vi "Autonics_Hall_GMR_Vector_report2014.vi"() -> ()   [LabVIEW 2018]
uses:
  <vilib>/Platform/NI_3dgraph.lvlib
  <vilib>/Utility/file.llb/Write To Spreadsheet File (DBL).vi
  <vilib>/DAQmx/create/channels.llb/DAQmx Create Channel (DO-Digital Output).vi
  <vilib>/DAQmx/write.llb/DAQmx Write (Digital 1D Bool 1Chan 1Samp).vi
  <vilib>/DAQmx/read.llb/DAQmx Read (Analog 2D DBL NChan NSamp).vi
  <vilib>/DAQmx/configure/timing.llb/DAQmx Timing (Sample Clock).vi
  <vilib>/DAQmx/create/channels.llb/DAQmx Create Channel (AI-Voltage-Basic).vi
  <resource>/objmgr/daqmx.rc
  <vilib>/Math Plots/3D Math Plots/3D Quiver/3D Quiver Datatype/3D Quiver Datatype.lvclass
  <vilib>/Math Plots/3D Math Plots/3D Quiver/3D Quiver Datatype/Public/Plot Helper (Vector).vi
  <vilib>/Analysis/Matrix/NI_Matrix.lvlib
  <vilib>/Utility/file.llb/Read From Spreadsheet File (DBL).vi
  <vilib>/Analysis/Matrix/Numeric/Multiply/Multiply - R,RM.vi
  <vilib>/Analysis/Matrix/Numeric/Multiply/Multiply - RM,R.vi
  <vilib>/Math Plots/2D Math Plots/2D Feather/2D Feather Datatype/2D Feather Datatype.lvclass
  <vilib>/Math Plots/2D Math Plots/2D Feather/2D Feather Datatype/Public/Plot Helper (Vector).vi
  <vilib>/Instr/_visa.llb/VISA Configure Serial Port (Instr).vi
  <vilib>/Math Plots/3D Math Plots/3D Quiver/3D Quiver XCtrl/3D Quiver.xctl
  <vilib>/Math Plots/2D Math Plots/2D Feather/2D Feather XCtrl/2D Feather.xctl
panel:
  out "2D Feather":refnum<class "2D Plot Datatype.lvclass">[](xcontrol)
  in  "GMR":refnum<k7>(container)
  in  "Z Length":dbl=2.0
  in  "X Length":dbl=50.0
  out "X_Z_Scale":sgl=111.11112
  in  "Invert ?":bool
  out "Time Step":u32
  in  "Open":bool
  out "3D Vector":refnum<class "3D Plot Datatype.lvclass">[](xcontrol)
  in  "Scan Distance":dbl=50.0
  in  "Multiplier":dbl=10.0
  in  "Save Button":bool
  in  "No Save":bool
  in  "Save/Open Link":path
  in  "ViewMode":i32(ring) items=["cwViewXYPlane", "cwViewXZPlane", "cwViewYZPlane", "cwViewUserDefined"]
  in  "Back data":bool
  in  "Data Type":u16(ring) items=["Normal", "dX", "dY"]
  in  "Scan Channel":fxp<+,8,8>
  in  "Scan Channel Control":tag="Dev3/port0/line0:7"
  in  "Sampling Rate(Hz)":dbl=15000.0
  in  "Samples per Channels":i32=1000
  in  "Min Volts":dbl=-10.0 format="%0.2f"
  in  "Max Volts":dbl=10.0 format="%0.2f"
  in  "Channels":tag="Dev3/ai0:63"
  in  "Scan Step (mm)":dbl=1.0
  in  "Scan":bool
  in  "Plot style":i32(ring)=5 items=["cwLine"=1, "cwPoint"=2, "cwLinePoint"=3, "cwHiddenLine"=4, "cwSurface"=5, "cwSurfaceLine"=6, "cwSurfaceNormal"=7, "cwContourLine"=8, "cwSurfaceContour"=9]
  in  "Hall":refnum<k7>(container)
  in  "Flow control":u16(ring) items=["None", "XON/XOFF", "RTS/CTS", "XON/XOFF & RTS/CTS", "DTR/DSR", "XON/XOFF & DTR/DSR"]
  in  "Stop bits":u16(ring)=10 items=["1.0"=10, "1.5"=15, "2.0"=20]
  in  "Parity":dbl
  in  "Data bits":u16=8 min=5 max=8 step=1
  in  "Baud Rate":u32=57600
  in  "COM Port":refnum<visa-resource-name>="COM3"
  in  "Travel per Pulse (mm)":dbl=0.002
  in  "Speed (mm/s)":dbl=5.0
  out "Current  Position (mm)":dbl format="%#_4g"
  in  "Move Distance (mm)":dbl=1.0
  in  "Stop Scan":bool
  in  "Stop":bool
  in  "Home":bool
  in  "Right":bool
  in  "Left":bool
  # "SCANER CONTROL"
  # "CRACKS INSPECTION"
  # "COM Setting"
  # "CHANNELS"
  # "TIMING"
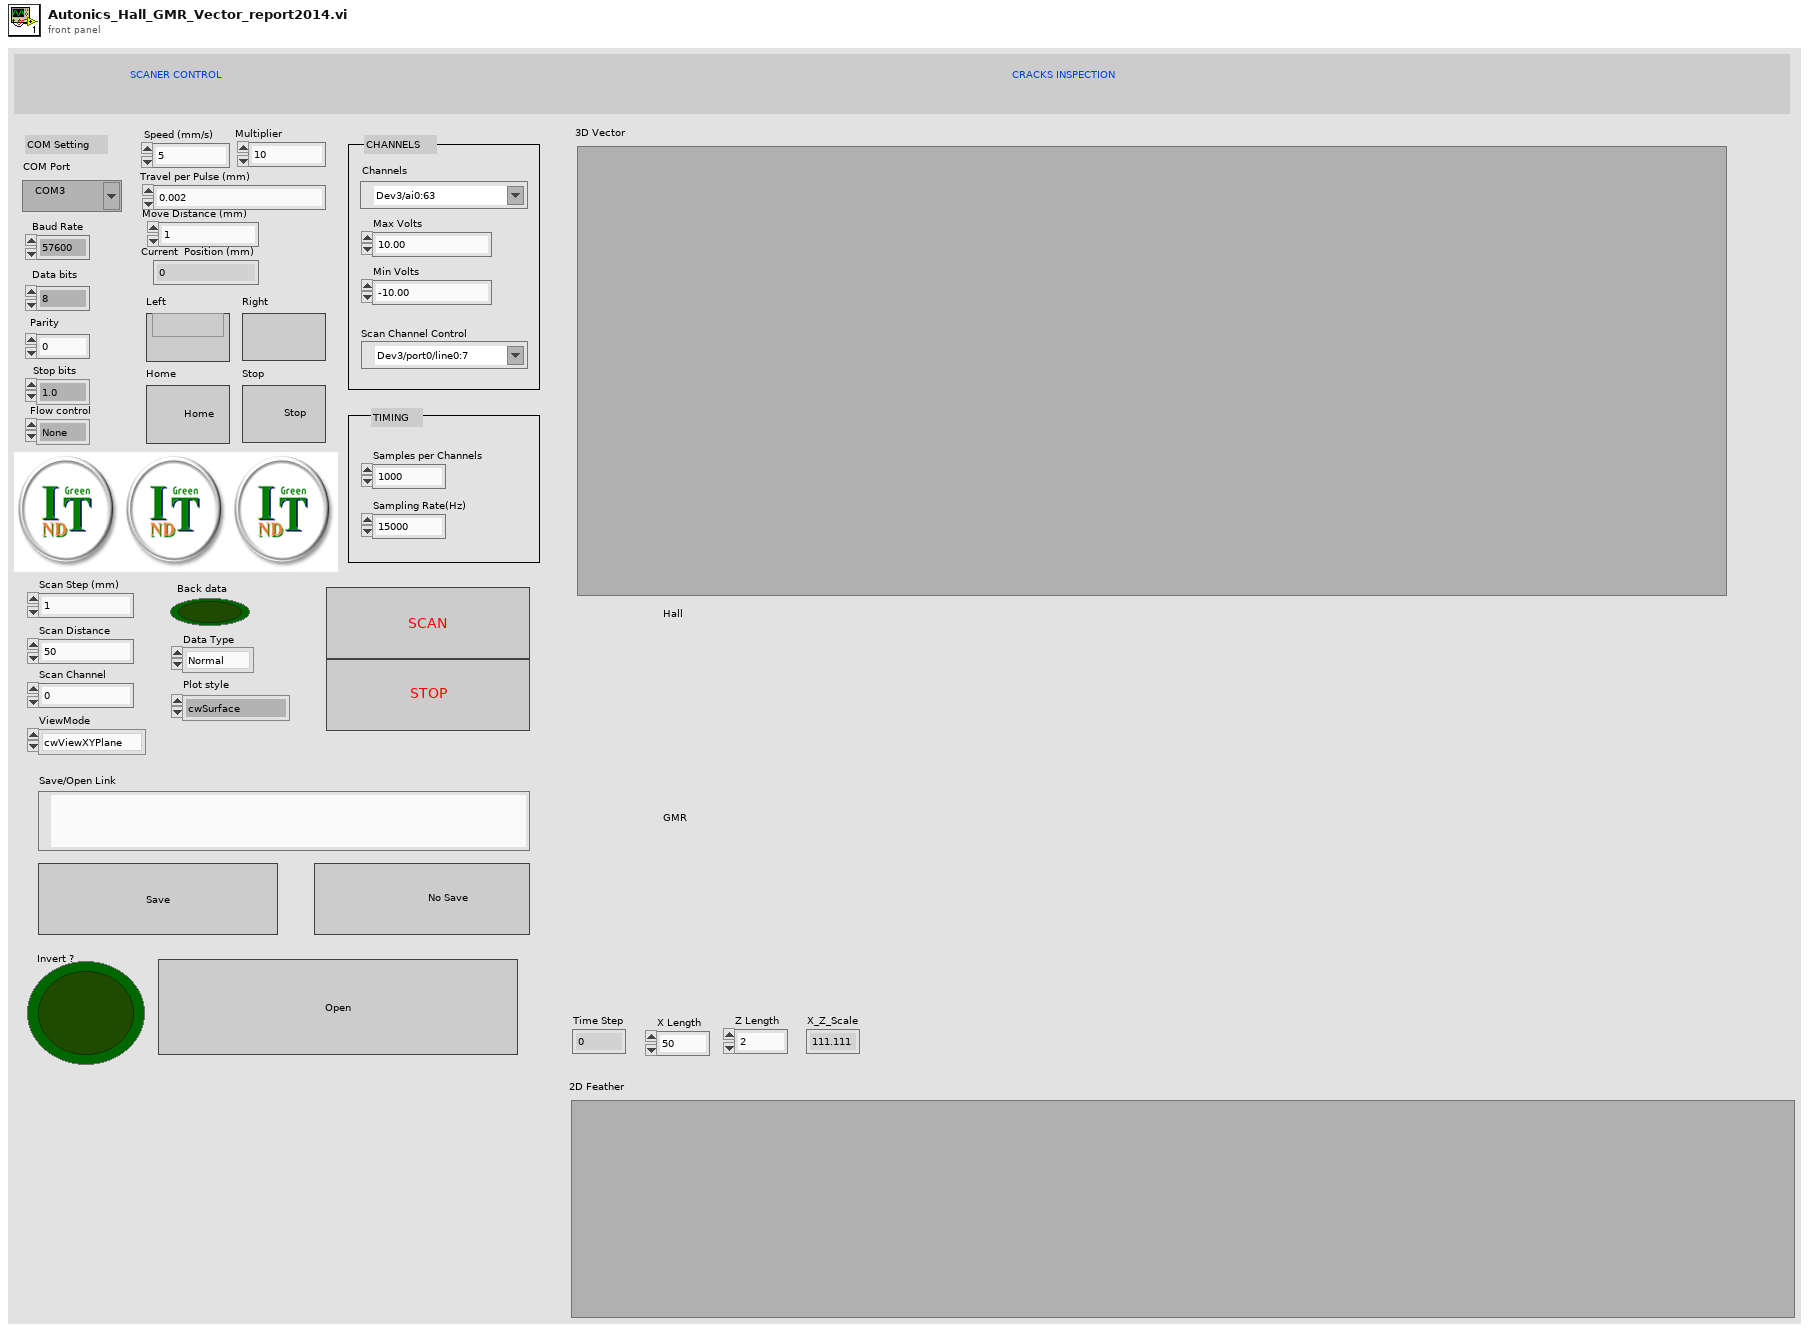
[diagram p1: front panel]
types:
  T1 = typedef "NI_Matrix.lvlib/RealMatrix.ctl" = dbl[][]
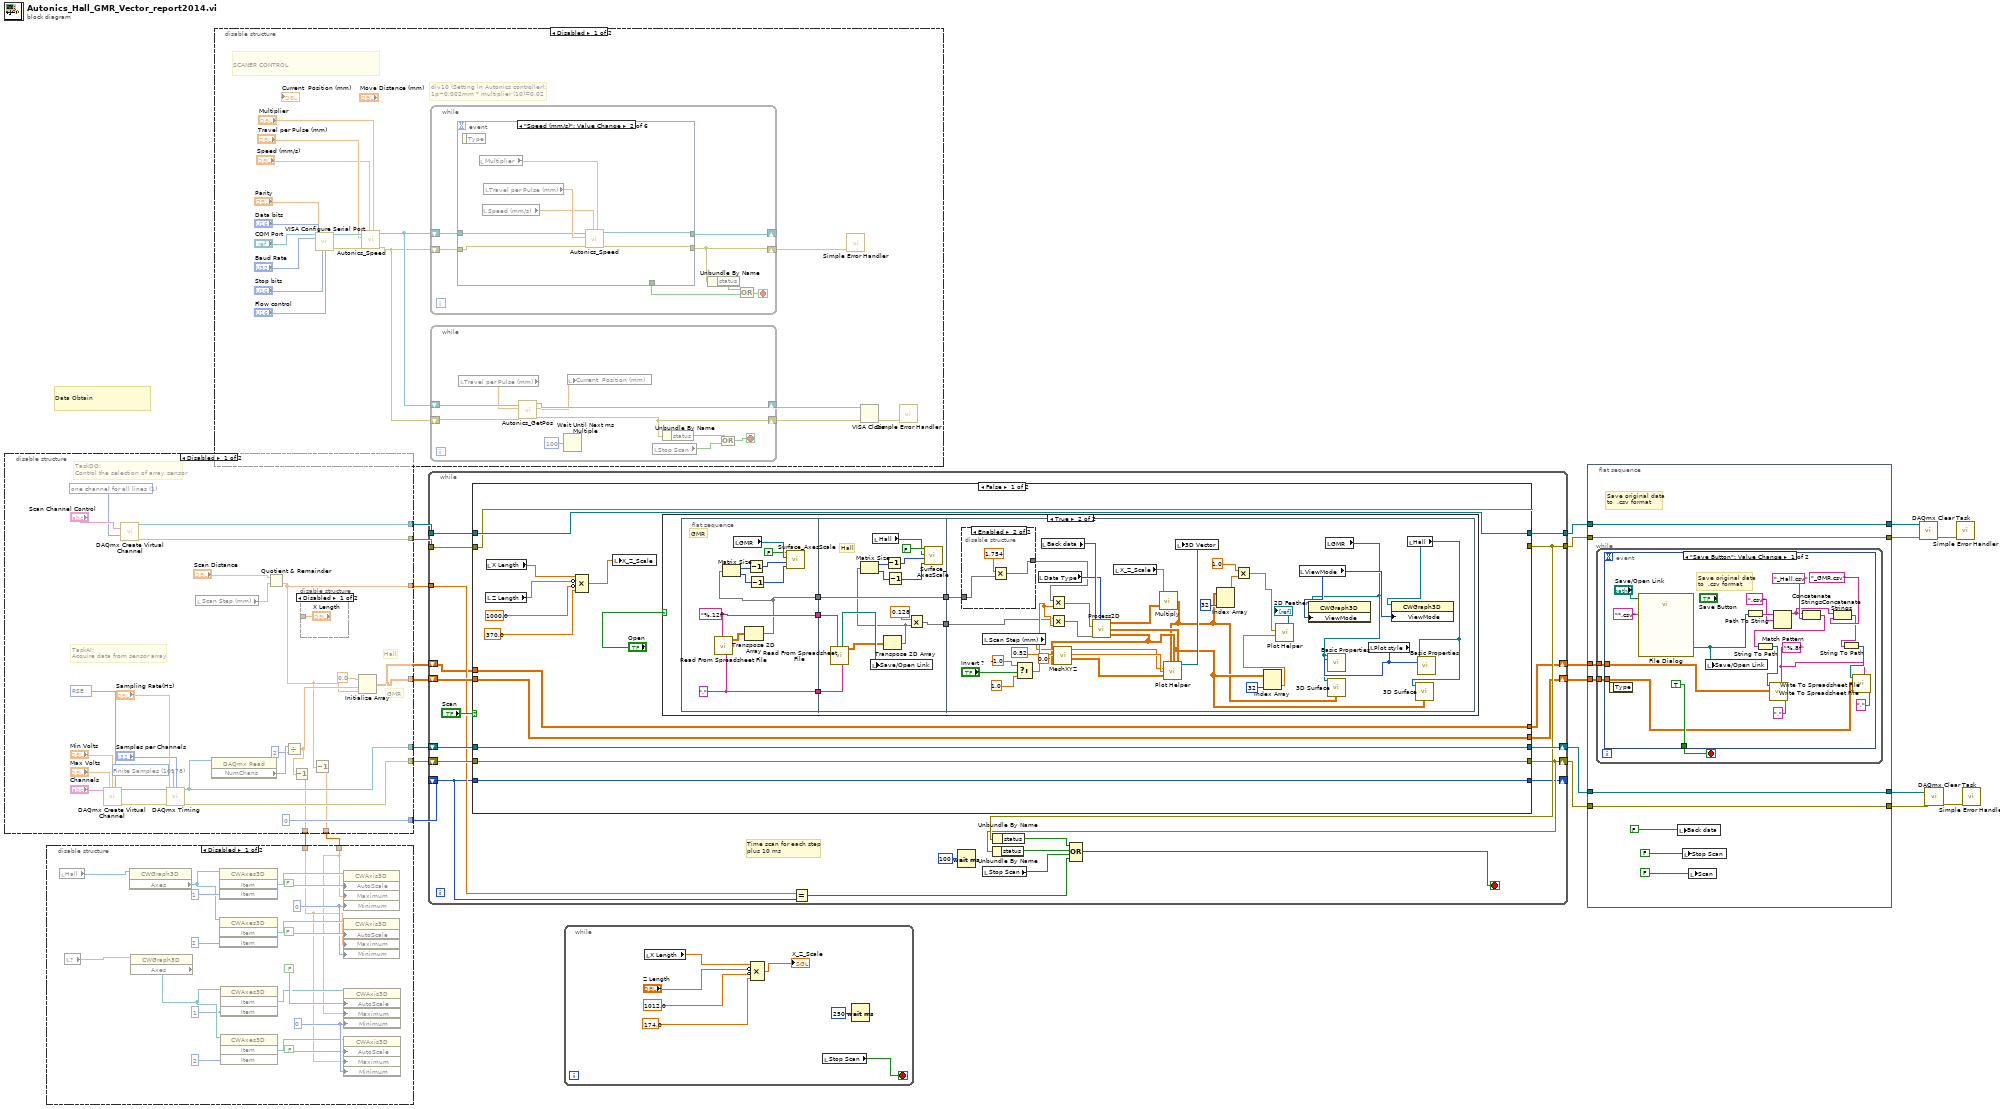
[diagram p0: block diagram]
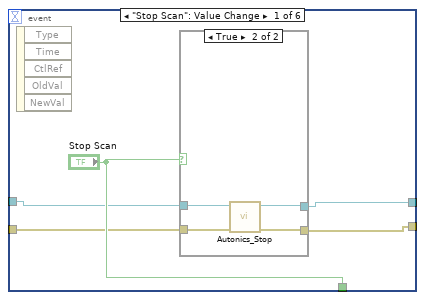
[diagram p5: hidden frame]
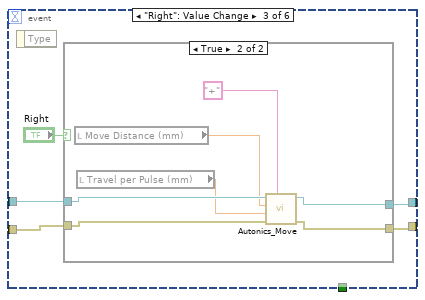
[diagram p7: hidden frame]
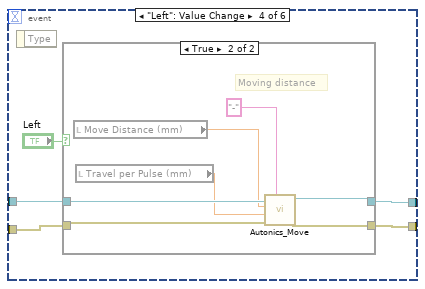
[diagram p9: hidden frame]
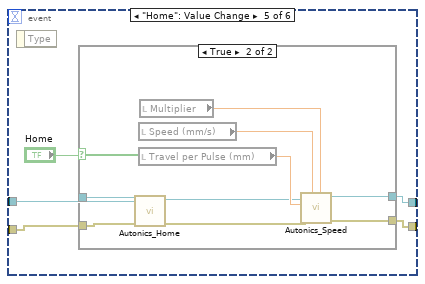
[diagram p11: hidden frame]
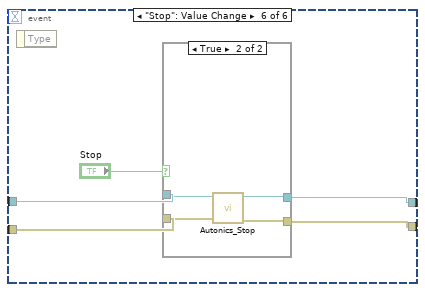
[diagram p13: hidden frame]
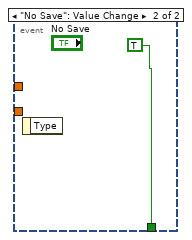
[diagram p16: hidden frame]
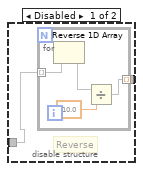
[diagram p18: hidden frame]
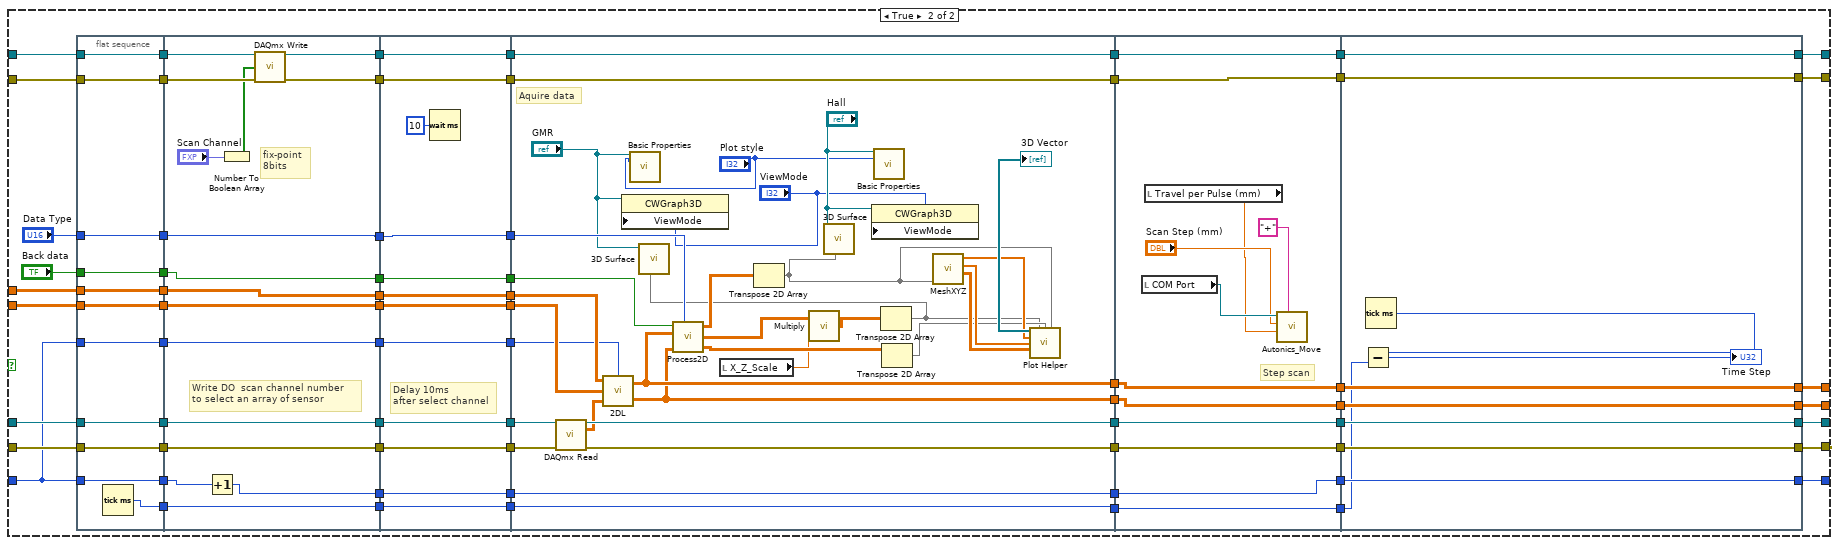
[diagram p19: hidden frame]
diagram:
  # "Data Obtain"
  n1 = disable-structure shown="Disabled" {
    disable-tunnel: [w47 _] -> w21
    disable-tunnel: [w44 _] -> w15
    disable-tunnel: [w43 _] -> w14
    disable-tunnel: [w41 _] -> w8
    disable-tunnel: [0 _] -> w7
    disable-tunnel: [w37 _] -> w6
    disable-tunnel: [w36 _] -> w4
    disable-tunnel: [w34 _] -> w3
    disable-tunnel: [w33 _] -> w2
    frame Disabled {
      w24 = 10083 items=["default"=-1, "RSE"=10083, "NRSE"=10078, "Differential"=10106, "Pseudodifferential"=12529] ("input terminal configuration")
      w25 = 10178 items=["Finite Samples"=10178, "Continuous Samples"=10123, "Hardware Timed Single Point"=12522] ("sample mode")
      w45 = 1 items=["one channel for each line", "one channel for all lines"] ("line grouping")
      # "TaskAI:\nAcquire data from sensor array"
      # "GMR"
      # "Hall"
      # "TaskDO: \nControl the selection of array sensor"
      n2 = call-poly <vilib>:"DAQmx Create Virtual Channel.vi"("maximum value"="Max Volts", "minimum value"="Min Volts", "input terminal configuration"=w24, "physical channels"="Channels") -> ("task out"=w32:refnum<k21>, "error out"=w31:errorcluster)  [unwired: 10 in]
      n3 = call-poly <vilib>:"DAQmx Create Virtual Channel.vi"("lines"="Scan Channel Control", "line grouping"=w45) -> ("task out"=w44:refnum<k21>, "error out"=w43:errorcluster)  [unwired: 12 in]
      n4 = call-poly <vilib>:"DAQmx Timing.vi"("task/channels in"=w32, "sample mode"=w25, "samples per channel"="Samples per Channels", "rate"="Sampling Rate(Hz)", "error in"=w31) -> ("task out"=w41:refnum<k21>, "error out"=w47:errorcluster)  [unwired: 9 in]
      n5 = local read "Scan Step (mm)"() -> (w40:dbl)
      n6 = property class="DAQmx Read"(reference=w41) -> ("NumChans"=w23:u32)  [unwired: 1 in, 2 out]
      n7 = Quotient & Remainder(x="Scan Distance", y=w40) -> (floor(x/y)=w33:dbl)  [unwired: 1 out]
      n8 = Divide(x=w23, y=u32 2) -> (x/y=w35:dbl)
      n9 = Decrement(x=w35) -> (x-1=w36:dbl)
      n10 = disable-structure shown="Disabled" {
        disable-tunnel: ["X Length" _] -> _
        frame Disabled {
        }
        frame Enabled {
        }
      }
      n11 = Decrement(x=w33) -> (x-1=w34:dbl)
      n12 = Initialize Array(0.0 ("element"), w35, w33) -> (w37:dbl[][])
    }
    frame Enabled {
    }
  }
  n13 = disable-structure shown="Disabled" {
    disable-tunnel: w4 -> [w50 _]
    disable-tunnel: w3 -> [w49 _]
    frame Disabled {
      w59 = 0
      w60 = 0
      n14 = local read "Hall"() -> (w68:refnum<k7>)
      n15 = local read item#-1() -> (w51)
      n16 = property class="CWGraph3D"(reference=w68) -> ("Axes"=w61:refnum<k7>)  [unwired: 1 in, 2 out]
      n17 = property class="CWGraph3D"(reference=w51) -> ("Axes"=w58:refnum<k7>)  [unwired: 1 in, 2 out]
      n18 = invoke class="CWAxes3D" method="Item"(reference=w61, "Item"=1) -> ("Item"=w67:refnum<k7>)  [unwired: 2 in, 3 out]
      n19 = invoke class="CWAxes3D" method="Item"(reference=w61, "Item"=2) -> ("Item"=w62:refnum<k7>)  [unwired: 2 in, 3 out]
      n20 = invoke class="CWAxes3D" method="Item"(reference=w58, "Item"=1) -> ("Item"=w52:refnum<k7>)  [unwired: 2 in, 3 out]
      n21 = invoke class="CWAxes3D" method="Item"(reference=w58, "Item"=2) -> ("Item"=w57:refnum<k7>)  [unwired: 2 in, 3 out]
      n22 = property class="CWAxis3D"(reference=w67, "AutoScale"=FALSE, "Maximum"=w49, "Minimum"=w60) -> ()  [unwired: 1 in, 2 out]
      n23 = property class="CWAxis3D"(reference=w62, "AutoScale"=FALSE, "Maximum"=w50, "Minimum"=w60) -> ()  [unwired: 1 in, 2 out]
      n24 = property class="CWAxis3D"(reference=w52, "AutoScale"=FALSE, "Maximum"=w49, "Minimum"=w59) -> ()  [unwired: 1 in, 2 out]
      n25 = property class="CWAxis3D"(reference=w57, "AutoScale"=FALSE, "Maximum"=w50, "Minimum"=w59) -> ()  [unwired: 1 in, 2 out]
    }
    frame Enabled {
    }
  }
  n26 = disable-structure shown="Disabled" {
    frame Disabled {
      # "div10 (Setting in Autonics controller):\n1p~0.002mm * multiplier (10)=0.02"
      # "SCANER CONTROL"
      n27 = call-poly "VISA Configure Serial Port"("VISA resource name"="COM Port", "baud rate (9600)"="Baud Rate", "data bits (8)"="Data bits", "parity (0:none)"="Parity", "stop bits (10: 1 bit)"="Stop bits", "flow control (0:none)"="Flow control") -> ("VISA resource name out"=w73:refnum<visa-resource-name>, "error out"=w72:errorcluster)  [unwired: 8 in]
      n28 = call "Autonics_Speed.vi"("Multiplier"="Multiplier", "Speed (mm/s)"="Speed (mm/s)", "error in (no error)"=w72, "Travel per  Pulse"="Travel per Pulse (mm)", "VISA resource name"=w73) -> ("error out"=w74:errorcluster, "VISA resource name out"=w75:refnum<visa-resource-name>)  [unwired: 5 in]
      n29 = while {
        shift-right: [w102] -> _
        shift-left: w75 -> [w101]
        shift-right: [w98] -> w78
        shift-left: w74 -> [w100]
        stop <- w97 stop-if-true
        n30 = event shown="[1] \"Speed (mm/s)\": Value Change" {
          selector: _ -> [_ _ _ _ _ _]
          dyn-events: _ -> [_ _ _ _ _ _]
          timeout: _ -> [_ _ _ _ _ _]
          tunnel: w101 -> [w106 w119 w123 w137 w153 w167]
          tunnel: w100 -> [w105 w118 w122 w136 w152 w166]
          tunnel: [w104 w117 w125 w139 w150 w169] -> w102
          tunnel: [w103 w116 w124 w138 w149 w168] -> w98
          tunnel: ["Stop Scan" _ _ _ _ _] -> w96
          event "Stop Scan": Value Change {
            n31 = event-data() -> ()  [unwired: 1 in, 5 out]
            n32 = case shown="True" "Stop Scan" {
              tunnel: [w109 w112] -> w104
              tunnel: [w108 w113] -> w103
              tunnel: w106 -> [w109 w111]
              tunnel: w105 -> [w108 w110]
              frame False {
              }
              frame True {
                n33 = call "Autonics_Stop.vi"("error in (no error)"=w110, "VISA resource name"=w111) -> ("error out"=w113:errorcluster, "VISA resource name out"=w112:refnum<visa-resource-name>)  [unwired: 8 in]
              }
            }
          }
          event "Speed (mm/s)": Value Change {
            n34 = event-data() -> ()  [unwired: 1 in, 1 out]
            n35 = local read "Multiplier"() -> (w114:dbl)
            n36 = local read "Speed (mm/s)"() -> (w115:dbl)
            n37 = local read "Travel per Pulse (mm)"() -> (w120:dbl)
            n38 = call "Autonics_Speed.vi"("Multiplier"=w114, "Speed (mm/s)"=w115, "error in (no error)"=w118, "Travel per  Pulse"=w120, "VISA resource name"=w119) -> ("error out"=w116:errorcluster, "VISA resource name out"=w117:refnum<visa-resource-name>)  [unwired: 5 in]
          }
          event "Right": Value Change {
            n39 = event-data() -> ()  [unwired: 1 in, 1 out]
            n40 = case shown="True" "Right" {
              tunnel: [w126 w132] -> w125
              tunnel: [w127 w131] -> w124
              tunnel: w123 -> [w126 w134]
              tunnel: w122 -> [w127 w133]
              frame False {
              }
              frame True {
                n41 = local read "Move Distance (mm)"() -> (w130:dbl)
                n42 = local read "Travel per Pulse (mm)"() -> (w129:dbl)
                n43 = call "Autonics_Move.vi"("Direction (+)"="+", "error in (no error)"=w133, "Travel per Pulse (mm)"=w129, "Move Distance (mm)"=w130, "VISA resource name"=w134) -> ("error out"=w131:errorcluster, "VISA resource name out"=w132:refnum<visa-resource-name>)  [unwired: 5 in]
              }
            }
          }
          event "Left": Value Change {
            n44 = event-data() -> ()  [unwired: 1 in, 1 out]
            n45 = case shown="True" "Left" {
              tunnel: [w141 w146] -> w139
              tunnel: [w140 w145] -> w138
              tunnel: w137 -> [w141 w148]
              tunnel: w136 -> [w140 w147]
              frame False {
              }
              frame True {
                # "Moving distance"
                n46 = local read "Move Distance (mm)"() -> (w143:dbl)
                n47 = local read "Travel per Pulse (mm)"() -> (w142:dbl)
                n48 = call "Autonics_Move.vi"("Direction (+)"="-", "error in (no error)"=w147, "Travel per Pulse (mm)"=w142, "Move Distance (mm)"=w143, "VISA resource name"=w148) -> ("error out"=w145:errorcluster, "VISA resource name out"=w146:refnum<visa-resource-name>)  [unwired: 5 in]
              }
            }
          }
          event "Home": Value Change {
            n49 = event-data() -> ()  [unwired: 1 in, 1 out]
            n50 = case shown="True" "Home" {
              tunnel: [w155 w157] -> w150
              tunnel: [w154 w156] -> w149
              tunnel: w153 -> [w155 w164]
              tunnel: w152 -> [w154 w163]
              frame False {
              }
              frame True {
                n51 = call "Autonics_Home.vi"("error in (no error)"=w163, "VISA resource name"=w164) -> ("error out"=w158:errorcluster, "VISA resource name out"=w159:refnum<visa-resource-name>)  [unwired: 8 in]
                n52 = local read "Speed (mm/s)"() -> (w161:dbl)
                n53 = local read "Travel per Pulse (mm)"() -> (w162:dbl)
                n54 = local read "Multiplier"() -> (w160:dbl)
                n55 = call "Autonics_Speed.vi"("Multiplier"=w160, "Speed (mm/s)"=w161, "error in (no error)"=w158, "Travel per  Pulse"=w162, "VISA resource name"=w159) -> ("error out"=w156:errorcluster, "VISA resource name out"=w157:refnum<visa-resource-name>)  [unwired: 5 in]
              }
            }
          }
          event "Stop": Value Change {
            n56 = event-data() -> ()  [unwired: 1 in, 1 out]
            n57 = case shown="True" "Stop" {
              tunnel: [w171 w172] -> w169
              tunnel: [w170 w175] -> w168
              tunnel: w167 -> [w171 w174]
              tunnel: w166 -> [w170 w173]
              frame False {
              }
              frame True {
                n58 = call "Autonics_Stop.vi"("error in (no error)"=w173, "VISA resource name"=w174) -> ("error out"=w175:errorcluster, "VISA resource name out"=w172:refnum<visa-resource-name>)  [unwired: 8 in]
              }
            }
          }
        }
        n59 = Unbundle By Name(w98) -> ("status"=w99:bool)
        n60 = Compound Arithmetic op=OR(w99, w96) -> (w97:bool)
      }
      n61 = while {
        shift-right: [w89] -> w77
        shift-left: w75 -> [w91]
        shift-right: [w88] -> w76
        shift-left: w74 -> [w90]
        stop <- w92 stop-if-true
        n62 = local read "Travel per Pulse (mm)"() -> (w87:dbl)
        n63 = call "Autonics_GetPos.vi"("error in (no error)"=w90, "Travel per Pulse (mm)"=w87, "VISA resource name"=w91) -> ("error out"=w88:errorcluster, "Current  Position (mm)"=w86:dbl, "VISA resource name out"=w89:refnum<visa-resource-name>)  [unwired: 6 in]
        n64 = Wait Until Next ms Multiple(millisecond multiple=u32 100) -> ()  [unwired: 1 out]
        n65 = local write "Current  Position (mm)"(w86) -> ()
        n66 = local read "Stop Scan"() -> (w93:bool)
        n67 = Unbundle By Name(w88) -> ("status"=w94:bool)
        n68 = Compound Arithmetic op=OR(w94, w93) -> (w92:bool)
      }
      n69 = call <vilib>:"Simple Error Handler.vi"("error in (no error)"=w78) -> ()  [unwired: 4 in, 5 out]
      n70 = VISA Close(VISA resource name=w77, error in (no error)=w76) -> (error out=w81:errorcluster)
      n71 = call <vilib>:"Simple Error Handler.vi"("error in (no error)"=w81) -> ()  [unwired: 4 in, 5 out]
    }
    frame Enabled {
    }
  }
  n72 = while {
    shift-right: [w177] -> w1
    shift-left: w6 -> [w196]
    shift-right: [w194] -> w19
    shift-left: w8 -> [w195]
    shift-right: [w186] -> w17
    shift-left: w21 -> [w197]
    tunnel: w15 -> [w190]
    tunnel: w14 -> [w189]
    tunnel: [w188] -> w12
    tunnel: [w187] -> w11
    shift-right: [w183] -> _
    shift-left: w7 -> [w181]
    tunnel: w2 -> [w182]
    shift-right: [w178] -> w5
    shift-left: w6 -> [w179]
    stop <- w193 stop-if-true
    # "Time scan for each step\nplus 10 ms"
    n73 = case shown="False" "Scan" {
      tunnel: w195 -> [w210 w347]
      tunnel: w197 -> [w209 w346]
      tunnel: w196 -> [w205 w345]
      tunnel: [w210 w342] -> w194
      tunnel: [w209 w341] -> w186
      tunnel: [w204 w308] -> w178
      tunnel: w190 -> [w208 w340]
      tunnel: w189 -> [w207 w339]
      tunnel: [w208 w336] -> w188
      tunnel: [w207 w335] -> w187
      tunnel: [w206 w318] -> w183
      tunnel: w181 -> [w206 w311]
      tunnel: w179 -> [w204 w312]
      tunnel: [w205 w306] -> w177
      frame False {
        n74 = local read "Z Length"() -> (w202:dbl)
        n75 = local read "X Length"() -> (w201:dbl)
        n76 = Compound Arithmetic op=MULTIPLY(w201, invert w202, invert 1000.0 ("value"), 370.0 ("value")) -> (w198:dbl)
        n77 = local write "X_Z_Scale"(w198) -> ()
        n78 = case shown="True" "Open" {
          frame False {
          }
          frame True {
            n79 = flat-sequence {
              tunnel: [w217] -> w214
              tunnel: [w225] -> w212
              tunnel: [w224] -> w211
              tunnel: [w239] -> w215
              tunnel: w214 -> [w239]
              tunnel: [w229] -> w213
              tunnel: w212 -> [w238]
              tunnel: w211 -> [w237]
              tunnel: w215 -> [w256]
              tunnel: w213 -> [w245]
              frame #0 {
                w225 = "," ("delimiter (\\t)")
                w224 = "%.12f" ("format (%.3f)")
                # "GMR"
                n80 = call-poly <vilib>:"Read From Spreadsheet File.vi"("delimiter (\\t)"=w225, "format (%.3f)"=w224) -> ("all rows"=w216:dbl[][])  [unwired: 5 in, 4 out]
                n81 = local read "GMR"() -> (w220:refnum<k7>)
                n82 = Transpose 2D Array(2D array=w216) -> (transposed array=w217:dbl[][])
                n83 = Matrix Size(0:w217) -> (1:w218:i32, 2:w222:i32)
                n84 = Decrement(x=w218) -> (x-1=w221:i32)
                n85 = Decrement(x=w222) -> (x-1=w223:i32)
                n86 = call "Surface_AxesScale.vi"("Y-axis Max"=w223, "X-axis max"=w221, "3D Surface"=w220, "Auto Scale"=FALSE) -> ()  [unwired: 8 in]
              }
              frame #1 {
                # "Hall"
                n87 = call-poly <vilib>:"Read From Spreadsheet File.vi"("delimiter (\\t)"=w238, "format (%.3f)"=w237) -> ("all rows"=w227:dbl[][], "new file path (Not A Path if cancelled)"=w236:path)  [unwired: 5 in, 3 out]
                n88 = local write "Save/Open Link"(w236) -> ()
                n89 = local read "Hall"() -> (w233:refnum<k7>)
                n90 = Transpose 2D Array(2D array=w227) -> (transposed array=w226:dbl[][])
                n91 = Matrix Size(0:w226) -> (1:w235:i32, 2:w231:i32)
                n92 = Decrement(x=w235) -> (x-1=w232:i32)
                n93 = Decrement(x=w231) -> (x-1=w230:i32)
                n94 = Multiply(x=0.128, y=w226) -> (x*y=w229:dbl[][])
                n95 = call "Surface_AxesScale.vi"("Y-axis Max"=w230, "X-axis max"=w232, "3D Surface"=w233, "Auto Scale"=FALSE) -> ()  [unwired: 8 in]
              }
              frame #2 {
                n96 = disable-structure shown="Enabled" {
                  disable-tunnel: w256 -> [w275 w282]
                  disable-tunnel: [w274 w281] -> w246
                  frame Disabled {
                    # "Reverse"
                    n97 = for {
                      tunnel: w275 -> [w279] mode=indexing
                      tunnel: [w276] -> w274 mode=indexing
                      n98 = Reverse 1D Array(array=w279) -> (reversed array=w277:dbl[])
                      n99 = Divide(x=w277, y=-10.0 ("t")) -> (x/y=w276:dbl[])
                    }
                  }
                  frame Enabled {
                    n100 = Multiply(x=1.754, y=w282) -> (x*y=w281:dbl[][])
                  }
                }
                n101 = local read "Scan Step (mm)"() -> (w259:dbl)
                n102 = Select(t=-1.0, s="Invert ?", f=1.0) -> (s? t:f=w267:dbl)
                n103 = local read "Data Type"() -> (w260:u16)
                n104 = local read "Back data"() -> (w261:bool)
                n105 = Multiply(x=w246, y=w267) -> (x*y=w254:dbl[][])
                n106 = Multiply(x=w245, y=w267) -> (x*y=w266:dbl[][])
                n107 = call "Process2D.vi"("Back Data"=w261, "Matrix X"=w254, "Matrix Y"=w266, "Data Type"=w260) -> ("Out Matrix X"=w243:T1, "Out Matrix Y"=w244:T1, "Out Matrix Z (zeros)"=w255:T1)  [unwired: 1 in]
                n108 = call "MeshXYZ.vi"("Input Matrix)"=w255, "Z- Lift-off"=0.0, "del Y"=0.52, "del X"=w259) -> ("Mesh Z (Matrix)"=w242:dbl[][], "Mesh Y (Array)"=w273:dbl[], "Mesh X (Array)"=w272:dbl[])  [unwired: 5 in]
                n109 = local read "X_Z_Scale"() -> (w257:sgl)
                n110 = call-poly <vilib>:"Multiply.vi"("Real Matrix A"=w243, "Real Scalar c"=w257) -> ("c * A"=w241:T1)
                n111 = call-poly <vilib>:"Plot Helper.vi"("Nx matrix"=w241, "Ny matrix"=w255, "Nz matrix"=w244, "x vector"=w272, "y vector"=w273, "z matrix"=w242) -> ("3D Plot lvclass Array out"=w271:refnum<class "3D Plot Datatype.lvclass">[])  [unwired: 3 in, 6 out]
                n112 = local write "3D Vector"(w271) -> ()
                n113 = Index Array(array=w241, index (col)=32 ("disabled index (col)")) -> (element=w248:dbl[])  [unwired: 1 in]
                n114 = Multiply(x=1.0, y=w248) -> (x*y=w247:dbl[])
                n115 = Index Array(array=w244, index (col)=32 ("disabled index (col)")) -> (element=w250:dbl[])  [unwired: 1 in]
                n116 = call-poly <vilib>:"Plot Helper.vi"("y vector"=w250, "x vector"=w247) -> ("2D Plot Class Obj Array out"=→"2D Feather":refnum<class "2D Plot Datatype.lvclass">[])  [unwired: 2 in, 7 out]
                n117 = local read "ViewMode"() -> (w264:i32)
                n118 = local read "GMR"() -> (w262:refnum<k7>)
                n119 = property class="CWGraph3D"(reference=w262, "ViewMode"=w264) -> ()  [unwired: 1 in, 2 out]
                n120 = call <vilib>:"3D Surface.vi"("z matrix"=w241, "3D graph"=w262) -> ()  [unwired: 8 in, 2 out]
                n121 = local read "Plot style"() -> (w265:i32)
                n122 = call <vilib>:"Basic Properties.vi"("3D graph"=w262, "plot style"=w265) -> ()  [unwired: 12 in, 2 out]
                n123 = local read "Hall"() -> (w263:refnum<k7>)
                n124 = property class="CWGraph3D"(reference=w263, "ViewMode"=w264) -> ()  [unwired: 1 in, 2 out]
                n125 = call <vilib>:"3D Surface.vi"("z matrix"=w244, "3D graph"=w263) -> ()  [unwired: 8 in, 2 out]
                n126 = call <vilib>:"Basic Properties.vi"("3D graph"=w263, "plot style"=w265) -> ()  [unwired: 12 in, 2 out]
              }
            }
          }
        }
      }
      frame True {
        n127 = flat-sequence {
          tunnel: w311 -> [w349]
          tunnel: w312 -> [w350]
          tunnel: w311 -> [w351]
          tunnel: "Data Type" -> [w352]
          tunnel: "Back data" -> [w353]
          tunnel: w339 -> [w354]
          tunnel: w340 -> [w355]
          tunnel: w345 -> [w356]
          tunnel: w346 -> [w357]
          tunnel: w347 -> [w358]
          tunnel: [w358] -> w304
          tunnel: [w357] -> w303
          tunnel: [w356] -> w302
          tunnel: [w355] -> w301
          tunnel: [w354] -> w300
          tunnel: [w353] -> w299
          tunnel: [w352] -> w298
          tunnel: [w351] -> w297
          tunnel: [w350] -> w296
          tunnel: [w349] -> w295
          tunnel: [w348] -> w291
          tunnel: [w374] -> w334
          tunnel: [w373] -> w332
          tunnel: [w372] -> w330
          tunnel: [w369] -> w328
          tunnel: [w368] -> w326
          tunnel: [w365] -> w322
          tunnel: [w364] -> w321
          tunnel: [w362] -> w315
          tunnel: [w361] -> w313
          tunnel: [w360] -> w310
          tunnel: w304 -> [w374]
          tunnel: w303 -> [w373]
          tunnel: w302 -> [w372]
          tunnel: w301 -> [w371]
          tunnel: w300 -> [w370]
          tunnel: w299 -> [w365]
          tunnel: w298 -> [w364]
          tunnel: w297 -> [w363]
          tunnel: w296 -> [w361]
          tunnel: w295 -> [w360]
          tunnel: [w359] -> w292
          tunnel: w291 -> [w359]
          tunnel: w334 -> [w386]
          tunnel: [w386] -> w333
          tunnel: w332 -> [w385]
          tunnel: [w385] -> w331
          tunnel: w330 -> [w384]
          tunnel: [w384] -> w329
          tunnel: w328 -> [w383]
          tunnel: [w383] -> w327
          tunnel: w326 -> [w382]
          tunnel: [w382] -> w325
          tunnel: [w380] -> w323
          tunnel: w322 -> [w380]
          tunnel: w321 -> [w379]
          tunnel: [w379] -> w319
          tunnel: [w378] -> w316
          tunnel: w315 -> [w378]
          tunnel: [w377] -> w314
          tunnel: w313 -> [w377]
          tunnel: w310 -> [w376]
          tunnel: [w376] -> w309
          tunnel: [w375] -> w293
          tunnel: w292 -> [w375]
          tunnel: [w416] -> w344
          tunnel: [w415] -> w343
          tunnel: w333 -> [w418]
          tunnel: w331 -> [w417]
          tunnel: w329 -> [w408]
          tunnel: [w414] -> w338
          tunnel: w327 -> [w414]
          tunnel: [w413] -> w337
          tunnel: w325 -> [w413]
          tunnel: w323 -> [w401]
          tunnel: w319 -> [w400]
          tunnel: [w411] -> w317
          tunnel: w316 -> [w411]
          tunnel: w314 -> [w409]
          tunnel: w309 -> [w407]
          tunnel: [w406] -> w307
          tunnel: [w405] -> w305
          tunnel: [w394] -> w294
          tunnel: w293 -> [w394]
          tunnel: w344 -> [w430]
          tunnel: w343 -> [w429]
          tunnel: w338 -> [w428]
          tunnel: w337 -> [w427]
          tunnel: w317 -> [w426]
          tunnel: w307 -> [w425]
          tunnel: w305 -> [w424]
          tunnel: w294 -> [w423]
          tunnel: [w430] -> w290
          tunnel: [w429] -> w289
          tunnel: [w428] -> w288
          tunnel: [w427] -> w287
          tunnel: [w426] -> w286
          tunnel: [w425] -> w285
          tunnel: [w424] -> w284
          tunnel: [w423] -> w283
          tunnel: [w434] -> w306
          tunnel: [w435] -> w308
          tunnel: [w436] -> w318
          tunnel: [w437] -> w335
          tunnel: [w438] -> w336
          tunnel: [w439] -> w341
          tunnel: [w440] -> w342
          tunnel: w290 -> [w440]
          tunnel: w289 -> [w439]
          tunnel: w288 -> [w438]
          tunnel: w287 -> [w437]
          tunnel: w286 -> [w436]
          tunnel: w285 -> [w435]
          tunnel: w284 -> [w434]
          tunnel: w283 -> [w432]
          frame #0 {
            n128 = Tick Count (ms)() -> (millisecond timer value=w348:u32)
          }
          frame #1 {
            # "fix-point\n8bits"
            # "Write DO  scan channel number\nto select an array of sensor"
            n129 = Increment(x=w363) -> (x+1=w362:i32)
            n130 = Number To Boolean Array(number="Scan Channel") -> (Boolean array=w366:bool[])
            n131 = call-poly <vilib>:"DAQmx Write.vi"("task/channels in"=w371, "data"=w366, "error in"=w370) -> ("task out"=w369:refnum<k21>, "error out"=w368:errorcluster)  [unwired: 10 in, 1 out]
          }
          frame #2 {
            # "Delay 10ms\nafter select channel"
            n132 = Wait (ms)(milliseconds to wait=u32 10) -> ()  [unwired: 1 out]
          }
          frame #3 {
            # "Aquire data"
            n133 = call-poly <vilib>:"DAQmx Read.vi"("task/channels in"=w418, "error in"=w417) -> ("task out"=w416:refnum<k21>, "data"=w410:dbl[][], "error out"=w415:errorcluster)  [unwired: 11 in]
            n134 = call "2DL.vi"("Insert Colum"=w407, "Input Matrix"=w410, "Input Array Y"=w408, "Input Array X"=w409) -> ("Out Array Y"=w405:dbl[][], "Out Array X"=w406:dbl[][])
            n135 = property class="CWGraph3D"(reference="GMR", "ViewMode"="ViewMode") -> ()  [unwired: 1 in, 2 out]
            n136 = call <vilib>:"Basic Properties.vi"("3D graph"="GMR", "plot style"="Plot style") -> ()  [unwired: 12 in, 2 out]
            n137 = call "Process2D.vi"("Back Data"=w401, "Matrix X"=w406, "Matrix Y"=w405, "Data Type"=w400) -> ("Out Matrix X"=w402:T1, "Out Matrix Y"=w390:T1, "Out Matrix Z (zeros)"=w404:T1)  [unwired: 1 in]
            n138 = local read "X_Z_Scale"() -> (w389:sgl)
            n139 = Transpose 2D Array(2D array=w402) -> (transposed array=w393:T1)
            n140 = call-poly <vilib>:"Multiply.vi"("Real Scalar c"=w389, "Real Matrix A"=w390) -> ("A * c"=w388:T1)
            n141 = call <vilib>:"3D Surface.vi"("z matrix"=w393, "3D graph"="Hall") -> ()  [unwired: 8 in, 2 out]
            n142 = property class="CWGraph3D"(reference="Hall", "ViewMode"="ViewMode") -> ()  [unwired: 1 in, 2 out]
            n143 = call <vilib>:"Basic Properties.vi"("3D graph"="Hall", "plot style"="Plot style") -> ()  [unwired: 12 in, 2 out]
            n144 = Transpose 2D Array(2D array=w388) -> (transposed array=w391:T1)
            n145 = call <vilib>:"3D Surface.vi"("z matrix"=w391, "3D graph"="GMR") -> ()  [unwired: 8 in, 2 out]
            n146 = Transpose 2D Array(2D array=w404) -> (transposed array=w392:T1)
            n147 = call "MeshXYZ.vi"("Input Matrix)"=w393) -> ("Mesh Z (Matrix)"=w399:dbl[][], "Mesh Y (Array)"=w398:dbl[], "Mesh X (Array)"=w397:dbl[])  [unwired: 8 in]
            n148 = call-poly <vilib>:"Plot Helper.vi"("Nx matrix"=w391, "Ny matrix"=w392, "Nz matrix"=w393, "x vector"=w397, "y vector"=w398, "z matrix"=w399) -> ("3D Plot lvclass Array out"=→"3D Vector":refnum<class "3D Plot Datatype.lvclass">[])  [unwired: 3 in, 6 out]
          }
          frame #4 {
            # "Step scan"
            n149 = local read "COM Port"() -> (w422:refnum<visa-resource-name>)
            n150 = local read "Travel per Pulse (mm)"() -> (w420:dbl)
            n151 = call "Autonics_Move.vi"("Direction (+)"="+", "Travel per Pulse (mm)"=w420, "Move Distance (mm)"="Scan Step (mm)", "VISA resource name"=w422) -> ()  [unwired: 6 in, 2 out]
          }
          frame #5 {
            n152 = Tick Count (ms)() -> (millisecond timer value=w433:u32)
            n153 = Subtract(x=w433, y=w432) -> (x-y=→"Time Step":u32)
          }
        }
      }
    }
    n154 = Equal?(x=w182, y=w181) -> (x = y?=w180:bool)
    n155 = Wait (ms)(milliseconds to wait=u32 100) -> ()  [unwired: 1 out]
    n156 = local read "Stop Scan"() -> (w191:bool)
    n157 = Unbundle By Name(w186) -> ("status"=w184:bool)
    n158 = Unbundle By Name(w187) -> ("status"=w185:bool)
    n159 = Compound Arithmetic op=OR(w185, w184, w191, w180) -> (w193:bool)
  }
  n160 = while {
    stop <- w441 stop-if-true
    n161 = local read "X Length"() -> (w447:dbl)
    n162 = Compound Arithmetic op=MULTIPLY(w447, invert "Z Length", invert 1012.0 ("value"), 174.0 ("value")) -> (→"X_Z_Scale":dbl)
    n163 = local read "Stop Scan"() -> (w441:bool)
    n164 = Wait (ms)(milliseconds to wait=u32 250) -> ()  [unwired: 1 out]
  }
  n165 = flat-sequence {
    tunnel: w19 -> [w456]
    tunnel: [w456] -> w18
    tunnel: w17 -> [w455]
    tunnel: [w455] -> w16
    tunnel: [w452] -> w10
    tunnel: w12 -> [w452]
    tunnel: [w451] -> w9
    tunnel: w11 -> [w451]
    tunnel: w5 -> [w450]
    tunnel: w1 -> [w448]
    frame #0 {
      # "Save original data\nto  .csv format"
      n166 = while {
        tunnel: w450 -> [w459]
        tunnel: w448 -> [w457]
        stop <- w458 stop-if-true
        n167 = event shown="[0] \"Save Button\": Value Change" {
          selector: _ -> [_ _]
          dyn-events: _ -> [_ _]
          timeout: _ -> [_ _]
          tunnel: w459 -> [w462 _]
          tunnel: [TRUE TRUE] -> w458
          tunnel: w457 -> [w461 _]
          event "Save Button": Value Change {
            w464 = "%.8f" ("format (%.3f)")
            # "Save original data\nto  .csv format"
            n168 = event-data() -> ()  [unwired: 1 in, 1 out]
            n169 = call "File Dialog"("start path"="Save/Open Link", "pattern (all files)"="*.csv") -> ("selected path"=w460:path)  [unwired: 10 in, 3 out]
            n170 = local write "Save/Open Link"(w460) -> ()
            n171 = Path To String(path=w460) -> (string=w473:string)
            n172 = Match Pattern(string=w473, regular expression=".csv") -> (before substring=w467:string)  [unwired: 1 in, 3 out]
            n173 = Concatenate Strings(w467, "_Hall.csv" ("format (%.3f)")) -> (w470:string)
            n174 = String To Path(string=w470) -> (path=w469:path)
            n175 = call-poly <vilib>:"Write To Spreadsheet File.vi"("delimiter (\\t)"="," ("delimiter (\\t)"), "format (%.3f)"=w464, "2D data"=w462, "file path (dialog if empty)"=w469) -> ()  [unwired: 4 in, 1 out]
            n176 = Concatenate Strings(w467, "_GMR.csv" ("format (%.3f)")) -> (w466:string)
            n177 = String To Path(string=w466) -> (path=w465:path)
            n178 = call-poly <vilib>:"Write To Spreadsheet File.vi"("delimiter (\\t)"="," ("delimiter (\\t)"), "format (%.3f)"=w464, "2D data"=w461, "file path (dialog if empty)"=w465) -> ()  [unwired: 4 in, 1 out]
          }
          event "No Save": Value Change {
            n179 = event-data() -> ()  [unwired: 1 in, 1 out]
          }
        }
      }
      n180 = local write "Back data"(FALSE ("Back data")) -> ()
      n181 = local write "Stop Scan"(FALSE ("Exit")) -> ()
      n182 = local write "Scan"(FALSE ("Scan")) -> ()
    }
  }
  n183 = call <vilib>:"DAQmx Clear Task.vi"("task in"=w10, "error in"=w9) -> ("error out"=w13:errorcluster)  [unwired: 13 in]
  n184 = call <vilib>:"DAQmx Clear Task.vi"("task in"=w18, "error in"=w16) -> ("error out"=w20:errorcluster)  [unwired: 13 in]
  n185 = call <vilib>:"Simple Error Handler.vi"("error in (no error)"=w13) -> ()  [unwired: 4 in, 5 out]
  n186 = call <vilib>:"Simple Error Handler.vi"("error in (no error)"=w20) -> ()  [unwired: 4 in, 5 out]
